vi "Add Glyph to Picture - Image.vi"(4 "Mask Color (Black)":u32(colorbox), 5 "Position (0,0)":cluster{"Horizontal":i16, "Vertical":i16}, 6 "Glyph {image}":T1, 7 "picture in":picture) -> (3 "picture out":picture)   [LabVIEW 2025, in "XNode Support.lvlib"]
doc: "Adds a glyph to an image at the specified point, interpreting the \"Mask Color\" as transparent.\nThe inputs of both the image in, and the glyph can be either a Picture, an Image Cluster, or a Pixmap."
uses:
  XNode Support.lvlib
  <vilib>/picture/picture.llb/imagedata.ctl
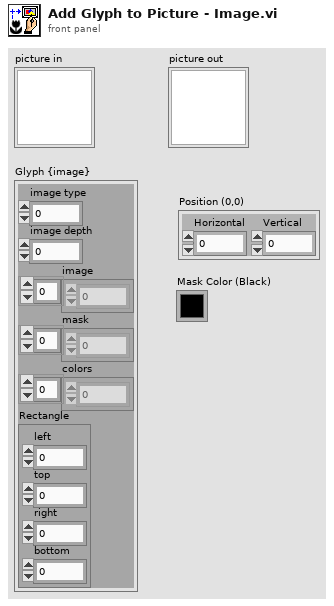
[diagram p1: front panel]
types:
  T1 = typedef "imagedata.ctl" = cluster{"image type":i32, "image depth":i32, "image":u8[], "mask":u8[], "colors":u32[], "Rectangle":cluster{"left":i16, "top":i16, "right":i16, "bottom":i16}}
  T2 = cluster{"Horizontal":i16, "Vertical":i16, "Horizontal":i16, "Vertical":i16}
  T3 = cluster{"left":i16, "top":i16, "right":i16, "bottom":i16}
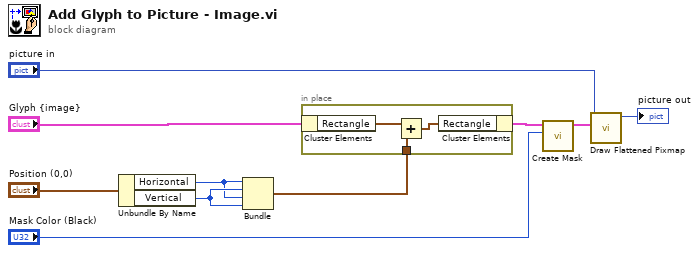
[diagram p0: block diagram]
diagram:
  n1 = Unbundle By Name("Position (0,0)") -> ("Horizontal"=w1:i16, "Vertical"=w6:i16)
  n2 = Bundle("Horizontal"=w1, "Vertical"=w6, "Horizontal"=w1, "Vertical"=w6) -> (w4:T2)  [unwired: 1 in]
  n3 = in-place {
    in-place-border: w4 -> [w11]
    n4 = in-place-cluster #1("Glyph {image}") -> ("Rectangle"=w13:T3)
    n5 = Add(x=w13, y=w11) -> (x+y=w12:cluster{i16, i16, i16, i16})
    n6 = in-place-cluster #1("Rectangle"=w12) -> (w10:T1)
  }
  n7 = call <vilib>:"Create Mask.vi"("Mask Color (Black)"="Mask Color (Black)", "image data"=w10) -> ("image data"=w8:T1)  [unwired: 9 in]
  n8 = call <vilib>:"Draw Flattened Pixmap.vi"("image data"=w8, "picture"="picture in") -> ("new picture"=→"picture out":picture)  [unwired: 7 in]
